vi "RT Main.vi"() -> ()   [LabVIEW 2013]
uses:
  <resource>/objmgr/ni.dex.rc
  <vilib>/Platform/TimedLoop/XDataNode/XDataNode.xnode
  <vilib>/Platform/TimedLoop/XDataNode/nitl_modes.ctl
  <vilib>/Platform/TimedLoop/XDataNode/XDNodeRunTimeDep.lvlib
  <vilib>/Platform/TimedLoop/XDataNode/wakeup.ctl
  <vilib>/Platform/TimedLoop/XDataNode/timing_clust.ctl
  <vilib>/rvi/interface/nirviOpenFPGA/nirviOpenFPGA.xnode
  <vilib>/myRIO/Instrument Drivers/Utilities/Utilities.lvlib
  <vilib>/rvi/interface/nirviReadWriteControl/nirviReadWriteControl.xnode
  <vilib>/rvi/interface/Simulation/niFpgaSimulationCallBeginRW.vi
  <vilib>/rvi/errors/niLvFpgaAdjustHostInterfaceError.vi
  <vilib>/rvi/interface/nirviCloseFPGA/nirviCloseFPGA.xnode
  NiFpgaLv.dll
  <vilib>/Utility/error.llb/Error Cluster From Error Code.vi
  <vilib>/FPGAPlugInAG/Dynamic/niLvFpga_Close_Dynamic.vi
  Program Files (x86)/National Instruments/LabVIEW 2013/ProjectTemplates/Source/myRIO/Dictaphone/myRIO v1.1/myRIO-1900 Customized FPGA.vi
panel:
  out "error out":errorcluster
  in  "Frequency Selector":T1(ring)
  out "End?":bool
  out "Connected?":bool
  in  "Stop":bool
  # "Overview: This sample project acquires audio data from the myRIO audio input channel, set the filter frequency band using the Frequency Selector, and generates the data on the audio output channel.  Both data sets are published using a network stream, which requires WiFi to be configured.\nRequirements: LabVIEW FPGA Module, Network Streams software on the NI myRIO RT target \nInstructions:\n1. Check the myRIO target IP Address in the project and make sure the target IP Address is correct. \n2. Connect a microphone to the audio input jack. Connect headphones or a speaker to the audio output jack.\n3. Run the VI and adjust the value of Frequency Selector."
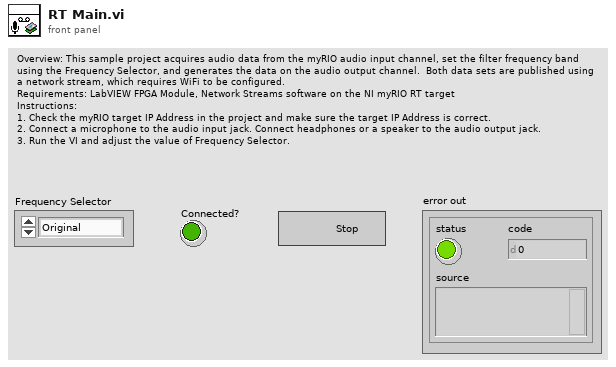
[diagram p1: front panel]
types:
  T1 = enum16{"Original", "< 500 Hz", "500 Hz - 1 kHz", "1 kHz - 2 kHz", "> 2 kHz"}
  T2 = typedef "XDNodeRunTimeDep.lvlib/timing_clust.ctl" = cluster{"Expected End [f-1]":u64, "Actual End [f-1]":u64, "Finished Late? [f-1]":bool, "Expected End [i-1]":u64, "Actual End [i-1]":u64, "Finished Late? [i-1]":bool, "Expected Start [i]":u64, "Actual Start [i]":u64, "Expected Start [f]":u64, "Actual Start [f]":u64, "Source Name":string, "Structure Name":string, "Period":i64, "Deadline":i64, "Offset":i64, "Start":i64, "Priority":i32, "Timeout":i32, "Mode":T3, "Wakeup Reason":T4, "Error":errorcluster, "Source Type":string, "Secondary Source Type":string, "Global End Time":u64, "Global Start Time":u64, "Frame Duration":u64, "Iteration Duration":u64, "Assigned CPU":i32, "I/O Scan Engine Mode":u32}
  T3 = typedef "XDNodeRunTimeDep.lvlib/nitl_modes.ctl" = enum32{"No Change", "Process missed periods, maintain original phase", "Discard missed periods, maintain original phase", "Process missed periods, ignore original phase", "Discard missed periods, ignore original phase"}
  T4 = typedef "XDNodeRunTimeDep.lvlib/wakeup.ctl" = enum32{"Normal", "Aborted", "Asynchronous wakeup", "Timing source error", "Timed loop error", "Timeout"}
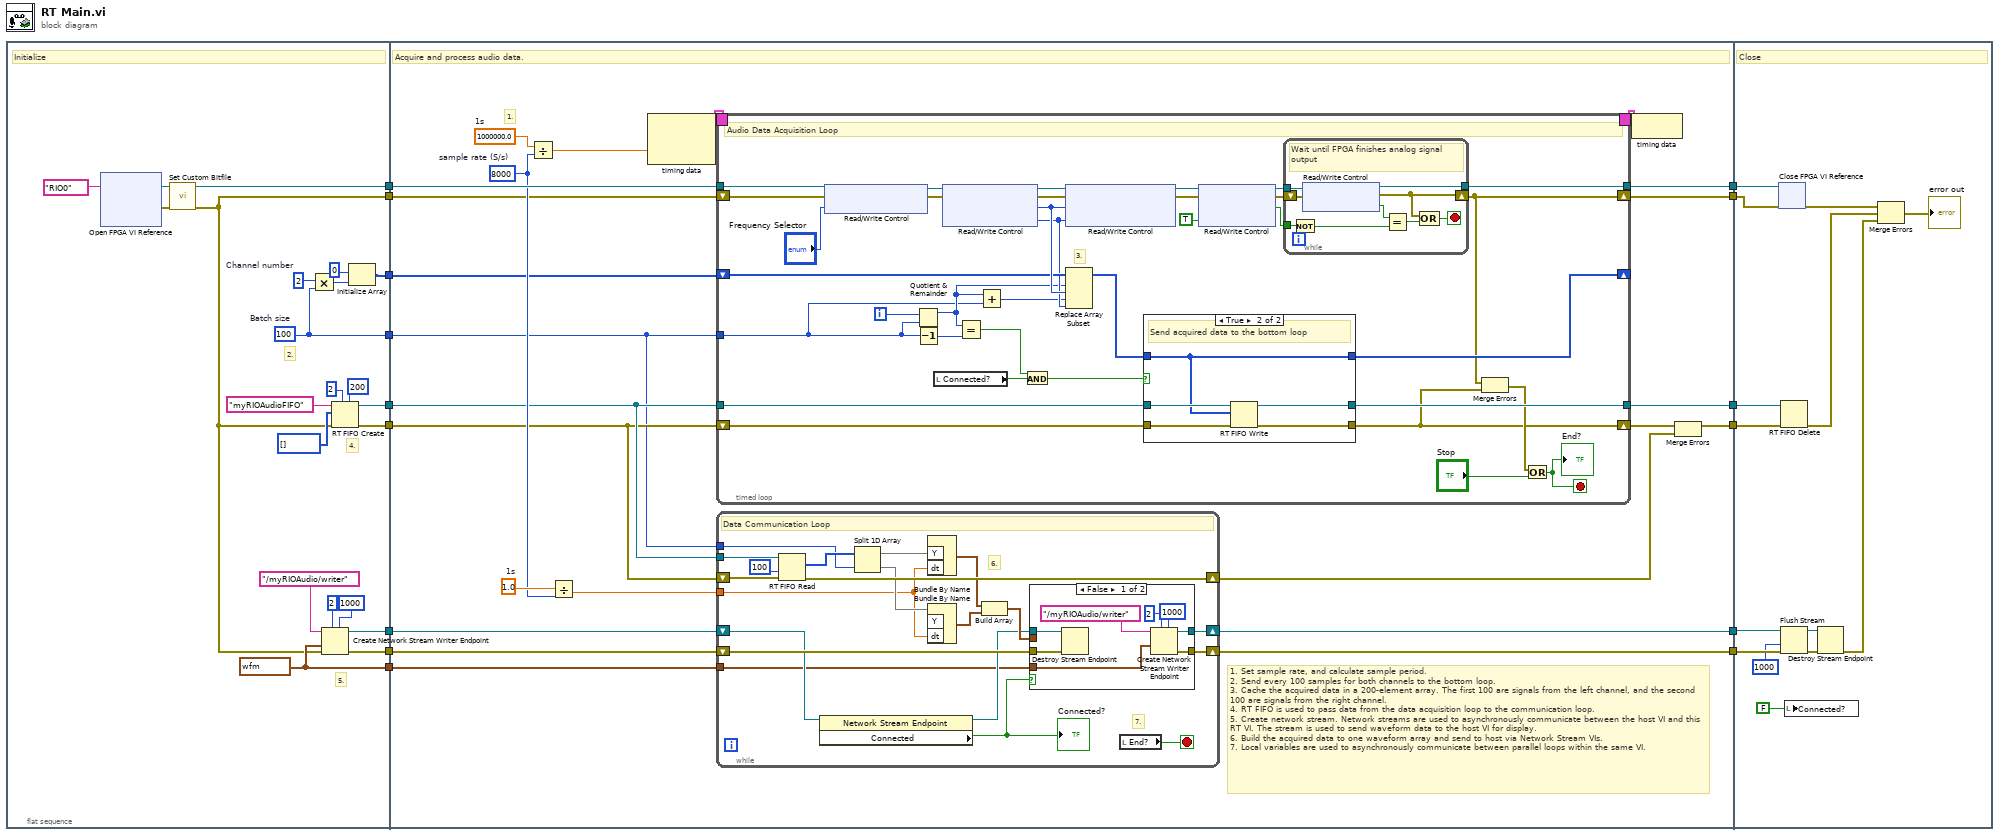
[diagram p0: block diagram]
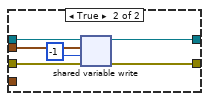
[diagram p3: hidden frame]
diagram:
  n1 = flat-sequence {
    tunnel: [w34] -> w11
    tunnel: [w21] -> w10
    tunnel: [w29] -> w7
    tunnel: [w28] -> w6
    tunnel: [w24] -> w5
    tunnel: [w23] -> w4
    tunnel: [w22] -> w3
    tunnel: [w17] -> w2
    tunnel: [w16] -> w1
    tunnel: [w60] -> w15
    tunnel: [w59] -> w14
    tunnel: [w46] -> w13
    tunnel: [w58] -> w12
    tunnel: w11 -> [w55]
    tunnel: w10 -> [w44]
    tunnel: [w54] -> w9
    tunnel: [w49] -> w8
    tunnel: w7 -> [w45]
    tunnel: w6 -> [w43]
    tunnel: w5 -> [w42]
    tunnel: w4 -> [w41]
    tunnel: w3 -> [w40]
    tunnel: w2 -> [w39]
    tunnel: w1 -> [w38]
    tunnel: w15 -> [w165]
    tunnel: w14 -> [w167]
    tunnel: w13 -> [w162]
    tunnel: w12 -> [w161]
    tunnel: w9 -> [w159]
    tunnel: w8 -> [w158]
    frame #0 {
      w17 = 100  # Batch size
      w19 = 2  # Channel number
      w24 = waveform(i16)[] [{"t0"=timestamp(0 s since 1904-01-01), "dt"=0.000125, "Y"=[0, 0, 0, 0, 0, 0, 0, 0, 0, 0, 0, 0, 0, 0, 0, 0, 0, 0, 0, 0, 0, 0, 0, 0, 0, 0, 0, 0, 0, 0, 0, 0, 0, 0, 0, 0, 0, 0, 0, 0, 0, 0, 0, 0, 0, 0, 0, 0, 0, 0, 0, 0, 0, 0, 0, 0, 0, 0, 0, 0, 0, 0, 0, 0, 0, 0, 0, 0, 0, 0, 0, 0, 0, 0, 0, 0, 0, 0, 0, 0, 0, 0, 0, 0, 0, 0, 0, 0, 0, 0, 0, 0, 0, 0, 0, 0, 0, 0, 0, 0]}, {"t0"=timestamp(0 s since 1904-01-01), "dt"=0.000125, "Y"=[0, 0, 0, 0, 0, 0, 0, 0, 0, 0, 0, 0, 0, 0, 0, 0, 0, 0, 0, 0, 0, 0, 0, 0, 0, 0, 0, 0, 0, 0, 0, 0, 0, 0, 0, 0, 0, 0, 0, 0, 0, 0, 0, 0, 0, 0, 0, 0, 0, 0, 0, 0, 0, 0, 0, 0, 0, 0, 0, 0, 0, 0, 0, 0, 0, 0, 0, 0, 0, 0, 0, 0, 0, 0, 0, 0, 0, 0, 0, 0, 0, 0, 0, 0, 0, 0, 0, 0, 0, 0, 0, 0, 0, 0, 0, 0, 0, 0, 0, 0]}]
      # "2."
      # "5."
      # "4."
      # "Initialize"
      n2 = xnode "Open FPGA VI Reference"("resource name"=tag "RIO0") -> ("FPGA VI Reference Out"=w36:refnum<k20>, "error out"=w35:errorcluster)  [unwired: 1 in]
      n3 = call <vilib>:"Set Custom Bitfile.vi"("error in (no error)"=w35, "Customized FPGA Reference in"=w36) -> ("error out"=w21:errorcluster, "Customized FPGA Reference out"=w34:refnum<k20>)  [unwired: 8 in]
      n4 = Multiply(x=w19, y=w17) -> (x*y=w20:i32)
      n5 = Create Network Stream Writer Endpoint(5:1000 ("timeout in ms (-1)"), 7:2 ("writer buffer size"), 8:w21, 9:w24, 11:"/myRIOAudio/writer" ("writer name")) -> (0:w23:errorcluster, 3:w22:refnum<k21>)  [unwired: 2 in]
      n6 = RT FIFO Create(0:"myRIOAudioFIFO" ("name (unnamed)"), 1:i16[] [], 3:w21, 4:u32 2 ("size (10)"), 6:u32 200 ("elements in array (1)")) -> (8:w29:refnum<k33>, 11:w28:errorcluster)  [unwired: 3 in, 1 out]
      n7 = Initialize Array(i16 0, w20) -> (w16:i16[])
    }
    frame #1 {
      w52 = 1.0  # 1s
      w61 = 1000000.0  # 1s
      w51 = 8000  # sample rate (S/s)
      # "1. Set sample rate, and calculate sample period.\n2. Send every 100 samples for both channels to the bottom loop.\n3. Cache the acquired data in a 200-element array. The first 100 are signals from the left channel, and the second 100 are signals from the right channel. \n4. RT FIFO is used to pass data from the data acquisition loop to the communication loop. \n5. Create network stream. Network streams are used to asynchronously communicate between the host VI and this RT VI. The stream is used to send waveform data to the host VI for display.\n6. Build the acquired data to one waveform array and send to host via Network Stream VIs.\n7. Local variables are used to asynchronously communicate between parallel loops within the same VI."
      # "1."
      # "Acquire and process audio data."
      n8 = Divide(x=w61, y=w51) -> (x/y=w53:dbl)
      n9 = Divide(x=w52, y=w51) -> (x/y=w50:dbl)
      n10 = node-c288(w53) -> (w57:T2)  [unwired: 1 in]
      n11 = timed-loop {
        tunnel: w45 -> [w94]
        tunnel: [w93] -> w58
        shift-right: [w62] -> w48
        shift-left: w43 -> [w92]
        timing: w57 -> [_]
        timing-out: [_] -> w56
        tunnel: w39 -> [w67]
        tunnel: w55 -> [w86]
        tunnel: [w76] -> w54
        shift-right: [w71] -> _
        shift-left: w38 -> [w72]
        shift-right: [w64] -> w49
        shift-left: w44 -> [w85]
        i -> [w91]
        stop <- w95 stop-if-true
        # "3."
        # "Audio Data Acquisition Loop"
        n12 = xnode "Read/Write Control"("FPGA VI Reference In"=w86, "error in"=w85, "Frequency Selector"="Frequency Selector") -> ("FPGA VI Reference Out"=w84:refnum<k20>, "error out"=w83:errorcluster)
        n13 = Quotient & Remainder(x=w91, y=w67) -> (x-y*floor(x/y)=w69:i32)  [unwired: 1 out]
        n14 = Decrement(x=w67) -> (x-1=w90:i32)
        n15 = local read "Connected?"() -> (w88:bool)
        n16 = xnode "Read/Write Control"("FPGA VI Reference In"=w84, "error in"=w83) -> ("FPGA VI Reference Out"=w82:refnum<k20>, "error out"=w81:errorcluster, "AI.AudioIn_L.VAL"=w74:i16, "AI.AudioIn_R.VAL"=w70:i16)
        n17 = Equal?(x=w69, y=w90) -> (x = y?=w89:bool)
        n18 = Add(x=w69, y=w67) -> (x+y=w68:i32)
        n19 = And(x=w89, y=w88) -> (x .and. y?=w87:bool)
        n20 = xnode "Read/Write Control"("FPGA VI Reference In"=w82, "error in"=w81, "AO.AudioOut_L.VAL"=w74, "AO.AudioOut_R.VAL"=w70) -> ("FPGA VI Reference Out"=w80:refnum<k20>, "error out"=w75:errorcluster)
        n21 = Replace Array Subset(array=w72, new element #1=w74, index #1=w69, new element #2=w70, index #2=w68) -> (w73:i16[])
        n22 = case shown="True" w87 {
          tunnel: w94 -> [w108 w113]
          tunnel: w92 -> [w107 w112]
          tunnel: [w108 w111] -> w93
          tunnel: [w107 w110] -> w62
          tunnel: w73 -> [w106 w109]
          tunnel: [w106 w109] -> w71
          frame False {
            # "Cache acquired data"
          }
          frame True {
            # "Send acquired data to the bottom loop"
            n23 = RT FIFO Write(0:w113, 1:w109, 3:w112) -> (8:w111:refnum<k33>, 11:w110:errorcluster)  [unwired: 2 in, 2 out]
          }
        }
        n24 = xnode "Read/Write Control"("FPGA VI Reference In"=w80, "error in"=w75, "AO.SYS.GO"=TRUE) -> ("FPGA VI Reference Out"=w78:refnum<k20>, "error out"=w77:errorcluster, "AO.SYS.STAT"=w65:bool)
        n25 = while {
          tunnel: w78 -> [w105]
          tunnel: w65 -> [w104]
          shift-right: [w99] -> w64
          shift-left: w77 -> [w101]
          tunnel: [w100] -> w76
          stop <- w97 stop-if-true
          # "Wait until FPGA finishes analog signal output"
          n26 = Not(x=w104) -> (.not. x?=w102:bool)
          n27 = xnode "Read/Write Control"("FPGA VI Reference In"=w105, "error in"=w101) -> ("FPGA VI Reference Out"=w100:refnum<k20>, "error out"=w99:errorcluster, "AO.SYS.STAT"=w103:bool)
          n28 = Equal?(x=w103, y=w102) -> (x = y?=w98:bool)
          n29 = Compound Arithmetic op=OR(w99, w98) -> (w97:bool)
        }
        n30 = Merge Errors(w64, w62) -> (w63:errorcluster)
        n31 = Or(x=w63, y="Stop") -> (x .or. y?=w95:bool)
        "End?" <- w95
      }
      n32 = while {
        tunnel: w45 -> [w134]
        shift-right: [w136] -> w59
        shift-left: w41 -> [w139]
        shift-right: [w135] -> w60
        shift-left: w40 -> [w138]
        shift-right: [w132] -> w47
        shift-left: w43 -> [w133]
        tunnel: w39 -> [w123]
        tunnel: w50 -> [w122]
        tunnel: w42 -> [w120]
        stop <- w137 stop-if-true
        # "6."
        # "7."
        # "Data Communication Loop"
        n33 = RT FIFO Read(0:w134, 2:100 ("timeout in ms (0)"), 3:w133) -> (9:w127:i16[], 11:w132:errorcluster)  [unwired: 1 in, 3 out]
        n34 = property class="Network Stream Endpoint"(reference=w138) -> (reference out=w128:refnum<k21>, "Connected"=w121:bool)  [unwired: 1 in, 1 out]
        "Connected?" <- w121
        n35 = Split 1D Array(array=w127, index=w123) -> (first subarray=w126:i16[], second subarray=w125:i16[])
        n36 = Bundle By Name("Y"=w126, "dt"=w122) -> (w131:waveform(i16))  [unwired: 1 in]
        n37 = Bundle By Name("Y"=w125, "dt"=w122) -> (w130:waveform(i16))  [unwired: 1 in]
        n38 = Build Array(w131, w130) -> (w129:waveform(i16)[])
        n39 = case shown="False" w121 {
          tunnel: w139 -> [w140 w153]
          tunnel: [w145 w152] -> w136
          tunnel: [w146 w151] -> w135
          tunnel: w129 -> [_ w149]
          tunnel: w128 -> [w141 w148]
          tunnel: w120 -> [w144 _]
          frame False {
            n40 = Destroy Stream Endpoint(8:w140, 11:w141) -> ()  [unwired: 1 out]
            n41 = Create Network Stream Writer Endpoint(5:1000 ("timeout in ms (-1)"), 7:2 ("writer buffer size"), 9:w144, 11:"/myRIOAudio/writer" ("writer name")) -> (0:w145:errorcluster, 3:w146:refnum<k21>)  [unwired: 3 in]
          }
          frame True {
            n42 = shared-variable-write(w148, w153, w149, -1 ("timeout ms (-1)")) -> (w151:refnum<k21>, w152:errorcluster)  [unwired: 1 out]
          }
        }
        n43 = local read "End?"() -> (w137:bool)
      }
      n44 = node-c288(w56) -> ()
      n45 = Merge Errors(w48, w47) -> (w46:errorcluster)
    }
    frame #2 {
      # "Close"
      n46 = xnode "Close FPGA VI Reference"("FPGA VI Reference In"=w159, "error in"=w158) -> ("error out"=w157:errorcluster)
      n47 = RT FIFO Delete(0:w161, 3:w162) -> (11:w156:errorcluster)  [unwired: 1 in]
      n48 = Flush Stream(8:w167, 9:1000 ("timeout in ms (-1)"), 11:w165) -> (0:w166:errorcluster, 3:w164:refnum<k21>)  [unwired: 1 in, 1 out]
      n49 = local write "Connected?"(FALSE ("Connected?")) -> ()
      n50 = Destroy Stream Endpoint(8:w166, 11:w164) -> (0:w155:errorcluster)
      n51 = Merge Errors(w157, w156, w155) -> (→"error out":errorcluster)
    }
  }
